vi "test Verify Multi Combos.vi"(8 "error in":errorcluster, 11 "Test Case In":refnum<class "LUnit Extensions Tests.lvclass">) -> (0 "error out":errorcluster, 3 "Test Case Out":refnum<class "LUnit Extensions Tests.lvclass">)   [LabVIEW 2020, in "LUnit Extensions Tests.lvclass"]
uses:
  LUnit Extensions Tests.lvclass
  C:/Program Files/National Instruments/LabVIEW 2026/vi.lib/Astemes/LUnit/Test Case.lvclass
  722a4156-14ed-4e4b-a2a1-892f914081a3.vi
  f4c42a0d-4aa0-4b67-bcd1-64490bc5ab90.vi
  b12c861c-1b8e-4e4d-838f-ddedcaafb5de.vi
  Source/Extensions/LUnit.Extension/LUnit.Extension.lvlib
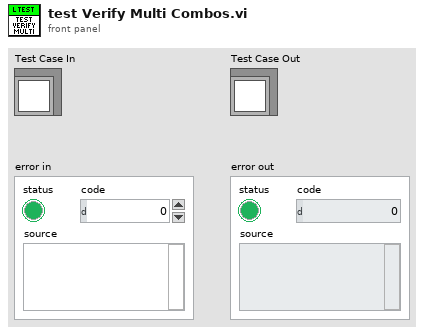
[diagram p1: front panel]
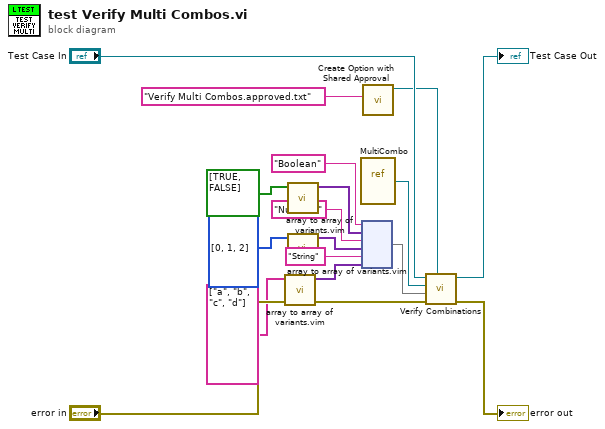
[diagram p0: block diagram]
diagram:
  n1 = call "array to array of variants.vim"("Array in"=string[] ["a", "b", "c", "d"]) -> ("Array out"=w7:variant[])  [unwired: 10 in]
  n2 = call "array to array of variants.vim"("Array in"=bool[] [TRUE, FALSE]) -> ("Array out"=w10:variant[])  [unwired: 10 in]
  n3 = call "array to array of variants.vim"("Array in"=i32[] [0, 1, 2]) -> ("Array out"=w8:variant[])  [unwired: 10 in]
  n4 = vi-ref "MultiCombo.vi"() -> (w4:refnum<vi>)
  n5 = node ("Build Map")("Boolean" ("key"), w10, "Numeric" ("key"), w8, "String" ("key"), w7) -> (w3:map{string, variant[]})
  n6 = call "Create Option with Shared Approval.vi"("Filename"="Verify Multi Combos.approved.txt") -> ("Options outs"=w1:refnum<class "Options.lvclass">)  [unwired: 10 in]
  n7 = call "Verify Combinations.vi"("Options"=w1, "error in"="error in", "ctl label -> value var[]"=w3, "VI in"=w4, "LUnit Test Case In"="Test Case In") -> ("error out"=→"error out":errorcluster, "LUnit Test Case Out"=→"Test Case Out":refnum<class "LUnit Extensions Tests.lvclass">)  [unwired: 5 in]
